vi "encoder_test_yaw.vi"() -> ()   [LabVIEW 2014]
uses:
  <vilib>/rvi/FXPMathLib/FxpSinAndCos/subVIs/nifxpmath_SinAndCos_SimConfig.ctl
  <vilib>/rvi/Emulation/niFpgaGetClockAttributes.vi
  <vilib>/rvi/Emulation/niFpgaSctlEmulationGetInTimedLoop.vi
  <vilib>/rvi/Emulation/niFpgaEmulationReportErrorSimple.vi
  <vilib>/rvi/eio/common/nirviEmuTemplateMethod_errors.vi
  <vilib>/rvi/Emulation/niFpgaProcessEmulError.vi
  <vilib>/rvi/Emulation/niFpgaCriticalErrorInLSC.vi
  <vilib>/rvi/FXPMathLib/FxpSinAndCos/simVIs/DllFxpSinAndCosTemp_sub.vi
  <vilib>/eio/EIONode/EIONode.xnode
  <vilib>/rvi/FXPMathLib/FxpMul/XNode/nifxpmath_Multiplier.xnode
  <vilib>/rvi/FXPMathLib/FxpSinAndCos/XNode/nifxpmath_SinAndCos.xnode
  <vilib>/rvi/FXPMathLib/sim/FxpSim.dll
panel:
  in  "Ini coe.":bool
  out "va":fxp<+/-,38,8>
  out "vb":fxp<+/-,38,8>
  in  "stop motor":bool
  in  "Fmr":fxp<+/-,21,11>
  out "vq_F":fxp<+/-,20,5> format="%.57g"
  out "vd_F":fxp<+/-,20,5>
  out "D_d (mm/s)":fxp<+/-,32,12>
  out "mt":u32
  out "omega (rad/s)":fxp<+/-,32,18>
  in  "mt0":u32
  out "D(mm)":fxp<+/-,22,7>
  out "rad(NrTheta)":fxp<+/-,33,18>
  out "Encoder Position":i32
  in  "Encoder Reset":bool
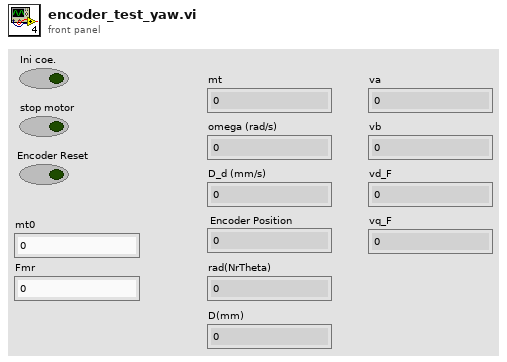
[diagram p1: front panel]
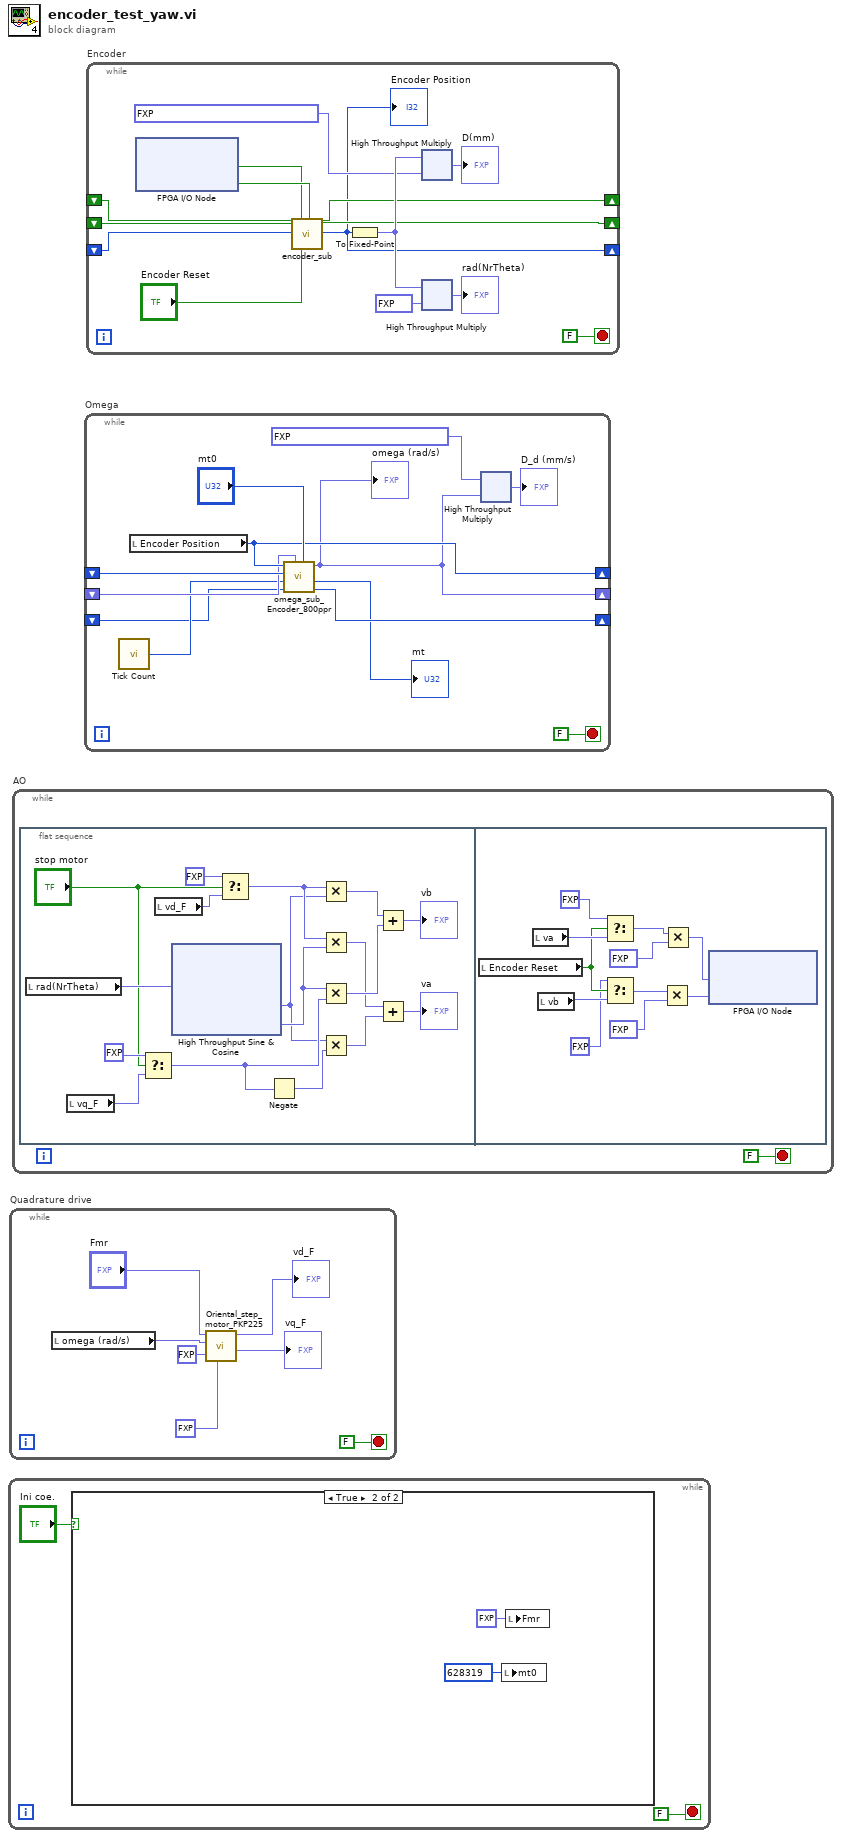
[diagram p0: block diagram]
diagram:
  n1 = while {
    stop <- FALSE stop-if-true
    n2 = case shown="True" "Ini coe." {
      frame False {
      }
      frame True {
        n3 = local write "mt0"(u32 628319 ("mt0")) -> ()
        n4 = local write "Fmr"(fxp<+/-,21,11> 50.0 ("Fmr")) -> ()
      }
    }
  }
  n5 = while "Quadrature drive" {
    stop <- FALSE stop-if-true
    n6 = local read "omega (rad/s)"() -> (w7:fxp<+/-,32,18>)
    n7 = call "Oriental_step_motor_PKP225.vi"("F_Threshold"=fxp<+,12,12> 10.0, "dFmr"=fxp<+/-,25,15> 0.0, "omega"=w7, "Fmr"="Fmr") -> ("vq_F"=→"vq_F":fxp<+/-,20,5>, "vd_F"=→"vd_F":fxp<+/-,20,5>)  [unwired: 6 in]
  }
  n8 = while "AO" {
    stop <- FALSE stop-if-true
    n9 = flat-sequence {
      frame #0 {
        n10 = local read "rad(NrTheta)"() -> (w28:fxp<+/-,33,18>)
        n11 = local read "vq_F"() -> (w26:fxp<+/-,20,5>)
        n12 = Select(t=fxp<+,20,5> 0.0, s="stop motor", f=w26) -> (s? t:f=w23:fxp<+/-,21,6>)
        n13 = local read "vd_F"() -> (w27:fxp<+/-,20,5>)
        n14 = xnode "High Throughput Sine & Cosine"("x (pi)"=w28) -> ("sin(x)"=w19:fxp<+/-,17,2>, "cos(x)"=w21:fxp<+/-,17,2>)
        n15 = Select(t=fxp<+,20,5> 0.0, s="stop motor", f=w27) -> (s? t:f=w20:fxp<+/-,21,6>)
        n16 = Negate(x=w23) -> (-x=w22:fxp<+/-,21,6>)
        n17 = Multiply(x=w20, y=w19) -> (x*y=w18:fxp<+/-,37,7>)
        n18 = Multiply(x=w20, y=w21) -> (x*y=w16:fxp<+/-,37,7>)
        n19 = Multiply(x=w21, y=w23) -> (x*y=w17:fxp<+/-,37,7>)
        n20 = Multiply(x=w19, y=w22) -> (x*y=w15:fxp<+/-,37,7>)
        n21 = Add(x=w18, y=w17) -> (x+y=→"vb":fxp<+/-,38,8>)
        n22 = Add(x=w16, y=w15) -> (x+y=→"va":fxp<+/-,38,8>)
      }
      frame #1 {
        n23 = local read "Encoder Reset"() -> (w62:bool)
        n24 = local read "va"() -> (w64:fxp<+/-,38,8>)
        n25 = local read "vb"() -> (w63:fxp<+/-,38,8>)
        n26 = Select(t=fxp<+/-,20,5> 5.0 ("y"), s=w62, f=w64) -> (s? t:f=w65:fxp<+/-,38,8>)
        n27 = Select(t=fxp<+/-,20,5> 0.0 ("y"), s=w62, f=w63) -> (s? t:f=w66:fxp<+/-,38,8>)
        n28 = Multiply(x=w66, y=fxp<+/-,20,5> -0.5) -> (x*y=w70:fxp<+/-,57,12>)
        n29 = Multiply(x=w65, y=fxp<+/-,20,5> -0.5) -> (x*y=w69:fxp<+/-,57,12>)
        n30 = xnode "FPGA I/O Node"("Mod8/AO2"=w69, "Mod8/AO3"=w70) -> ()  [unwired: 2 in, 2 out]
      }
    }
  }
  n31 = while "Omega" {
    shift-right: [w80] -> _
    shift-left: _ -> [w81]
    shift-right: [w73] -> _
    shift-left: _ -> [w79]
    shift-right: [w76] -> _
    shift-left: _ -> [w77]
    stop <- FALSE stop-if-true
    n32 = call "Tick Count"() -> ("Tick Count(Ticks)"=w78:u32)
    n33 = local read "Encoder Position"() -> (w80:i32)
    n34 = call "omega_sub_Encoder_800ppr.vi"("mt0"="mt0", "omega_pre"=w79, "ticks_m_pre"=w77, "ticks"=w78, "count_pre"=w81, "count"=w80) -> ("ticks_m"=w76:u32, "mt"=→"mt":u32, "omega"=w73:fxp<+/-,20,9>)  [unwired: 3 in]
    "omega (rad/s)" <- w73
    n35 = xnode ("High Throughput Multiply")("x"=fxp<+/-,26,1> 0.3183099031448364, "y"=w73) -> ("x*y"=→"D_d (mm/s)":fxp<+/-,46,10>)
  }
  n36 = while "Encoder" {
    shift-right: [w89] -> _
    shift-left: _ -> [w91]
    shift-right: [w88] -> _
    shift-left: _ -> [w90]
    shift-right: [w86] -> _
    shift-left: _ -> [w87]
    stop <- FALSE stop-if-true
    n37 = xnode "FPGA I/O Node"() -> ("Mod4/DI0"=w96:bool, "Mod4/DI1"=w97:bool)  [unwired: 2 in, 2 out]
    n38 = call "encoder_sub.vi"("A_pre"=w91, "B_pre"=w90, "Encoder Position_pre"=w87, "A input"=w96, "Encoder Position Reset"="Encoder Reset", "B input"=w97) -> ("A"=w89:bool, "B"=w88:bool, "Encoder Position (Counts)"=w86:i32)  [unwired: 19 in]
    "Encoder Position" <- w86
    n39 = To Fixed-Point(number=w86) -> (fixed-point=w94:fxp<+/-,32,32>)  [unwired: 1 in]
    n40 = xnode ("High Throughput Multiply")("x"=w94, "y"=fxp<+/-,24,0> 0.002499997615814209) -> ("x*y"=→"D(mm)":fxp<+/-,56,32>)
    n41 = xnode ("High Throughput Multiply")("x"=w94, "y"=fxp<+/-,24,0> 0.125) -> ("x*y"=→"rad(NrTheta)":fxp<+/-,56,32>)
  }
